vi "Launch BFECC.vi"(8 "error in (no error)":errorcluster, 11 "BFECC in":refnum<class "BFECC.lvclass">) -> (0 "error out":errorcluster, 3 "BFECC out":refnum<class "BFECC.lvclass">)   [LabVIEW 2018, in "BFECC.lvlib" / "BFECC.lvclass"]
doc: "Launch BFECC. MUST be used after a test (.tst) has been provided to the class private member."
uses:
  BFECC.lvclass
  BFECC.lvclass/BFECC.ctl
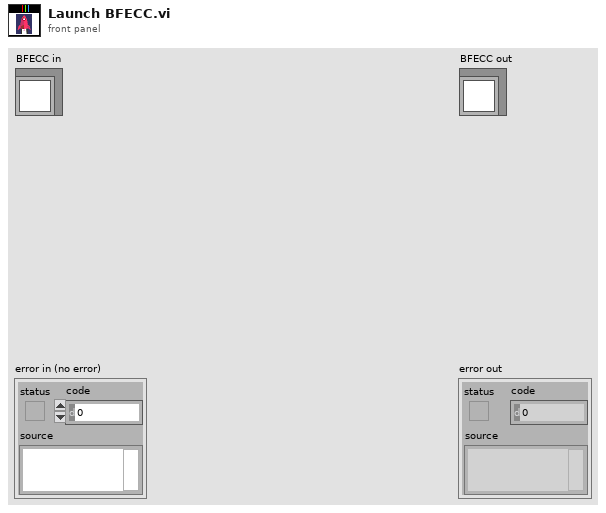
[diagram p1: front panel]
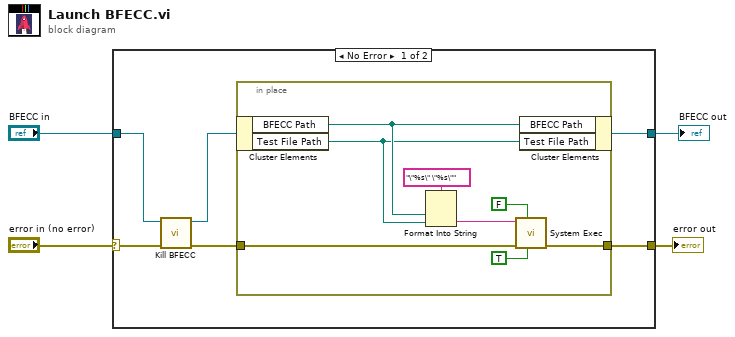
[diagram p0: block diagram]
diagram:
  n1 = case shown="No Error" "error in (no error)" {
    selector: "error in (no error)" -> [w8 w20]
    tunnel: [w10 w20] -> w3
    tunnel: [w9 w19] -> w1
    tunnel: "BFECC in" -> [w6 w19]
    frame No Error {
      n2 = call "Kill BFECC.vi"("error in (no error)"=w8, "BFECC in"=w6) -> ("error out"=w7:errorcluster, "BFECC out"=w5:refnum<class "BFECC.lvclass">)  [unwired: 8 in]
      n3 = in-place {
        in-place-border: w7 -> [w15]
        in-place-border: [w14] -> w10
        n4 = in-place-cluster #1(w5) -> ("BFECC Path"=w18:path, "Test File Path"=w17:path)
        n5 = Format Into String(format string="\"%s\" \"%s\"", w18, w17) -> (resulting string=w16:string)  [unwired: 2 in, 1 out]
        n6 = call <vilib>:"System Exec.vi"("run minimized? (F)"=TRUE, "wait until completion? (T)"=FALSE, "error in (no error)"=w15, "command line"=w16) -> ("error out"=w14:errorcluster)  [unwired: 4 in, 3 out]
        n7 = in-place-cluster #1("BFECC Path"=w18, "Test File Path"=w17) -> (w9:refnum<class "BFECC.lvclass">)
      }
    }
    frame Error {
    }
  }
  "error out" <- w3
  "BFECC out" <- w1
